vi "Digital Index To String.vi"(11 "Digital Index":i32) -> (3 "String":string)   [LabVIEW 2013, in "PMU Recorder Light.lvlib" / "Statnett C37.118 DLL.lvclass"]
uses:
  Statnett C37.118 DLL.lvclass
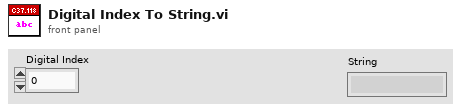
[diagram p1: front panel]
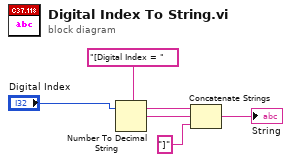
[diagram p0: block diagram]
diagram:
  n1 = Number To Decimal String(number="Digital Index") -> (decimal integer string=w5:string)  [unwired: 1 in]
  n2 = Concatenate Strings("[Digital Index = " ("string"), w5, "]" ("string")) -> (→"String":string)
